vi "Test_LocalQueue Handshake.vi"() -> ()   [LabVIEW 2013]
uses:
  Connection/auth -- cluster.ctl
  <vilib>/LabVIEW Open Source Project/Unicity/RandomStringGenerator/RandomStringGenerator.lvclass
  Connection/Connection.lvclass
panel:
  out "State verfied":bool
  out "Echo":string
  out "Echo verfied":bool
  out "Auth Ack/Nack":string
  out "Challenge verified":bool
  out "error out 2":errorcluster
  out "error out":errorcluster
  out "Client Reader":string
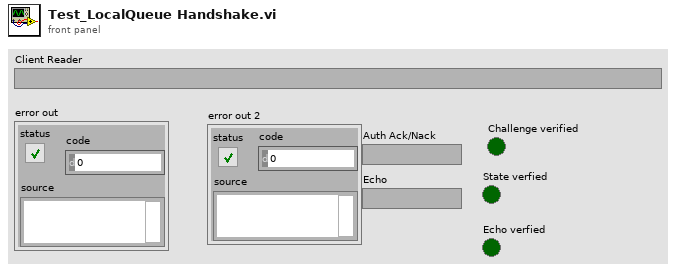
[diagram p1: front panel]
types:
  T1 = typedef "Connection_GOSPL.lvlib/Connection.lvclass/auth -- cluster.ctl" = cluster{"URL":string, "username":string, "state":string}
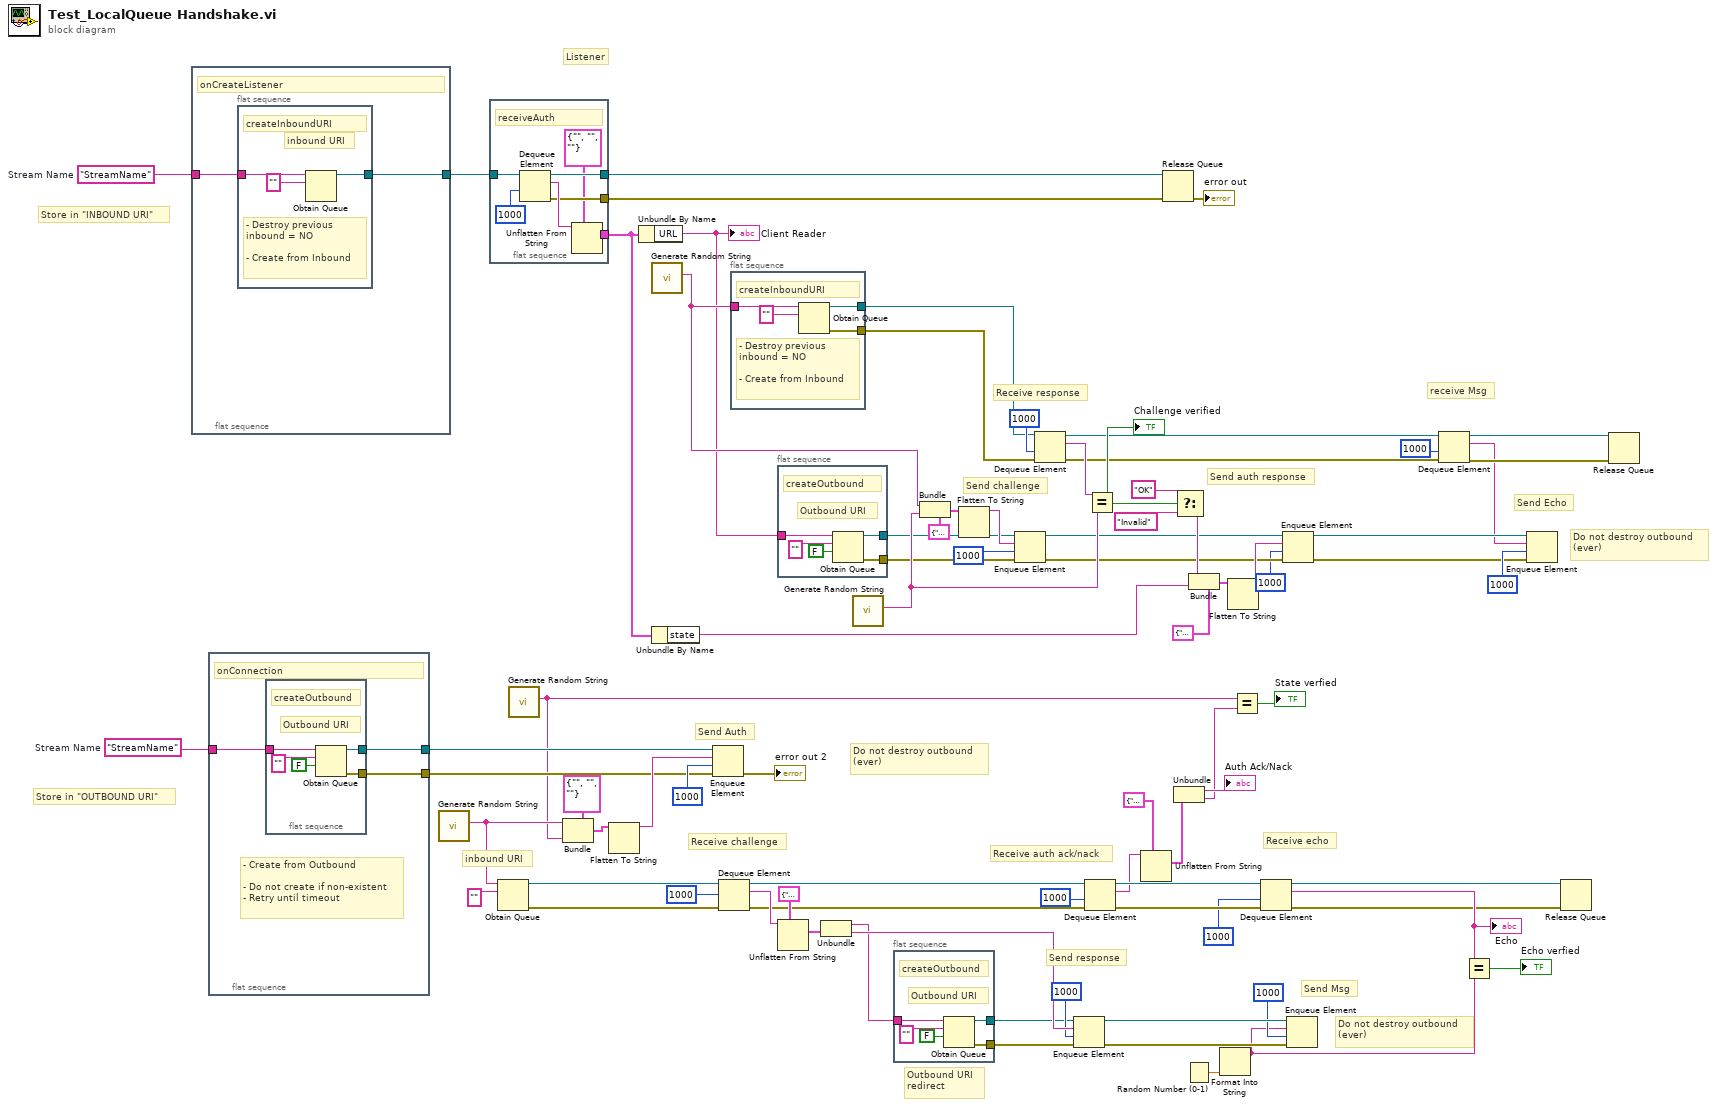
[diagram p0: block diagram]
diagram:
  w59 = "StreamName"  # Stream Name
  w64 = "StreamName"  # Stream Name
  # "Send Msg"
  # "receive Msg"
  # "Store in \"OUTBOUND URI\""
  # "Store in \"INBOUND URI\""
  # "Do not destroy outbound\n(ever)"
  # "Do not destroy outbound\n(ever)"
  # "Do not destroy outbound\n(ever)"
  # "inbound URI"
  # "Listener"
  # "Outbound URI\nredirect"
  # "Send Echo"
  # "Receive echo"
  # "Receive auth ack/nack"
  # "Send auth response"
  # "Receive response"
  # "Send response"
  # "Receive challenge"
  # "Send challenge"
  # "Send Auth"
  n1 = flat-sequence {
    tunnel: w64 -> [w84]
    tunnel: [w83] -> w63
    frame #0 {
      # "onCreateListener"
      n2 = flat-sequence {
        tunnel: w84 -> [w87]
        tunnel: [w85] -> w83
        frame #0 {
          # "- Destroy previous\ninbound = NO\n\n- Create from Inbound"
          # "inbound URI"
          # "createInboundURI"
          n3 = Obtain Queue(name (unnamed)=w87, element data type="") -> (queue out=w85:refnum<queue>)  [unwired: 3 in, 2 out]
        }
      }
    }
  }
  n4 = flat-sequence {
    tunnel: w59 -> [w90]
    tunnel: [w89] -> w56
    tunnel: [w88] -> w53
    frame #0 {
      # "- Create from Outbound\n\n- Do not create if non-existent\n- Retry until timeout"
      # "onConnection"
      n5 = flat-sequence {
        tunnel: w90 -> [w95]
        tunnel: [w93] -> w89
        tunnel: [w92] -> w88
        frame #0 {
          # "Outbound URI"
          # "createOutbound"
          n6 = Obtain Queue(name (unnamed)=w95, element data type="", create if not found? (T)=FALSE) -> (queue out=w93:refnum<queue>, error out=w92:errorcluster)  [unwired: 2 in, 1 out]
        }
      }
    }
  }
  n7 = call <vilib>:"Generate Random String.vi"() -> ("Random String"=w57:string)  [unwired: 11 in]
  n8 = flat-sequence {
    tunnel: [w102] -> w8
    tunnel: w63 -> [w101]
    tunnel: [w98] -> w62
    tunnel: [w97] -> w60
    frame #0 {
      # "receiveAuth"
      n9 = Dequeue Element(queue=w101, timeout in ms (-1)=1000) -> (queue out=w98:refnum<queue>, element=w99:string, error out=w97:errorcluster)  [unwired: 1 in, 1 out]
      n10 = Unflatten From String(type=T1 {"URL"="", "username"="", "state"=""} ("Authorization"), binary string=w99) -> (value=w102:T1)  [unwired: 3 in, 2 out]
    }
  }
  n11 = Obtain Queue(name (unnamed)=w57, element data type="") -> (queue out=w52:refnum<queue>, error out=w50:errorcluster)  [unwired: 3 in, 1 out]
  n12 = call <vilib>:"Generate Random String.vi"() -> ("Random String"=w12:string)  [unwired: 11 in]
  n13 = Bundle(cluster=T1 {"URL"="", "username"="", "state"=""} ("Authorization"), "URL"=w57, "state"=w12) -> (w73:T1)  [unwired: 1 in]
  n14 = Flatten To String(anything=w73) -> (data string=w55:string)  [unwired: 3 in, 2 out]
  n15 = Unbundle By Name(w8) -> ("URL"=w3:string)
  "Client Reader" <- w3
  n16 = call <vilib>:"Generate Random String.vi"() -> ("Random String"=w10:string)  [unwired: 11 in]
  n17 = Unbundle By Name(w8) -> ("state"=w7:string)
  n18 = Enqueue Element(queue=w56, element=w55, timeout in ms (-1)=1000, error in (no error)=w53) -> (error out=→"error out 2":errorcluster)  [unwired: 2 out]
  n19 = Dequeue Element(queue=w52, timeout in ms (-1)=1000, error in (no error)=w50) -> (queue out=w48:refnum<queue>, element=w49:string, error out=w47:errorcluster)  [unwired: 1 out]
  n20 = flat-sequence {
    tunnel: w10 -> [w106]
    tunnel: [w104] -> w11
    tunnel: [w103] -> w9
    frame #0 {
      # "- Destroy previous\ninbound = NO\n\n- Create from Inbound"
      # "createInboundURI"
      n21 = Obtain Queue(name (unnamed)=w106, element data type="") -> (queue out=w104:refnum<queue>, error out=w103:errorcluster)  [unwired: 3 in, 1 out]
    }
  }
  n22 = flat-sequence {
    tunnel: w3 -> [w111]
    tunnel: [w109] -> w2
    tunnel: [w108] -> w1
    frame #0 {
      # "Outbound URI"
      # "createOutbound"
      n23 = Obtain Queue(name (unnamed)=w111, element data type="", create if not found? (T)=FALSE) -> (queue out=w109:refnum<queue>, error out=w108:errorcluster)  [unwired: 2 in, 1 out]
    }
  }
  n24 = Unflatten From String(type=cluster{"redirect":string, "challenge":string} {"redirect"="", "challenge"=""} ("cluster"), binary string=w49) -> (value=w80:cluster{"redirect":string, "challenge":string})  [unwired: 3 in, 2 out]
  n25 = Unbundle(w80) -> ("redirect"=w6:string, "challenge"=w37:string)
  n26 = call <vilib>:"Generate Random String.vi"() -> ("Random String"=w74:string)  [unwired: 11 in]
  n27 = flat-sequence {
    tunnel: w6 -> [w116]
    tunnel: [w114] -> w5
    tunnel: [w113] -> w4
    frame #0 {
      # "Outbound URI"
      # "createOutbound"
      n28 = Obtain Queue(name (unnamed)=w116, element data type="", create if not found? (T)=FALSE) -> (queue out=w114:refnum<queue>, error out=w113:errorcluster)  [unwired: 2 in, 1 out]
    }
  }
  n29 = Bundle(cluster=cluster{"redirect":string, "challenge":string} {"redirect"="", "challenge"=""}, "redirect"=w10, "challenge"=w74) -> (w82:cluster{"redirect":string, "challenge":string})
  n30 = Flatten To String(anything=w82) -> (data string=w23:string)  [unwired: 3 in, 2 out]
  n31 = Enqueue Element(queue=w2, element=w23, timeout in ms (-1)=1000, error in (no error)=w1) -> (queue out=w21:refnum<queue>, error out=w16:errorcluster)  [unwired: 1 out]
  n32 = Dequeue Element(queue=w11, timeout in ms (-1)=1000, error in (no error)=w9) -> (queue out=w28:refnum<queue>, element=w29:string, error out=w24:errorcluster)  [unwired: 1 out]
  n33 = Enqueue Element(queue=w5, element=w37, timeout in ms (-1)=1000, error in (no error)=w4) -> (queue out=w35:refnum<queue>, error out=w32:errorcluster)  [unwired: 1 out]
  n34 = Dequeue Element(queue=w48, timeout in ms (-1)=1000, error in (no error)=w47) -> (queue out=w46:refnum<queue>, element=w41:string, error out=w45:errorcluster)  [unwired: 1 out]
  n35 = Equal?(x=w29, y=w74) -> (x = y?=w79:bool)
  "Challenge verified" <- w79
  n36 = Unflatten From String(type=cluster{"response":string, "header":string} {"response"="", "header"=""} ("cluster"), binary string=w41) -> (value=w68:cluster{"response":string, "header":string})  [unwired: 3 in, 2 out]
  n37 = Release Queue(queue=w62, error in (no error)=w60) -> (error out=→"error out":errorcluster)  [unwired: 1 in, 2 out]
  n38 = Unbundle(w68) -> ("response"=→"Auth Ack/Nack":string, "header"=w66:string)
  n39 = Select(t="OK", s=w79, f="Invalid") -> (s? t:f=w70:string)
  n40 = Random Number (0-1)() -> (number: 0 to 1=w33:dbl)
  n41 = Bundle(cluster=cluster{"response":string, "header":string} {"response"="", "header"=""}, "response"=w70, "header"=w7) -> (w71:cluster{"response":string, "header":string})
  n42 = Format Into String(w33) -> (resulting string=w31:string)  [unwired: 3 in, 1 out]
  n43 = Flatten To String(anything=w71) -> (data string=w17:string)  [unwired: 3 in, 2 out]
  n44 = Equal?(x=w12, y=w66) -> (x = y?=→"State verfied":bool)
  n45 = Dequeue Element(queue=w46, timeout in ms (-1)=1000, error in (no error)=w45) -> (queue out=w40:refnum<queue>, element=w44:string, error out=w39:errorcluster)  [unwired: 1 out]
  "Echo" <- w44
  n46 = Enqueue Element(queue=w21, element=w17, timeout in ms (-1)=1000, error in (no error)=w16) -> (queue out=w19:refnum<queue>, error out=w14:errorcluster)  [unwired: 1 out]
  n47 = Enqueue Element(queue=w35, element=w31, timeout in ms (-1)=1000, error in (no error)=w32) -> ()  [unwired: 3 out]
  n48 = Dequeue Element(queue=w28, timeout in ms (-1)=1000, error in (no error)=w24) -> (queue out=w26:refnum<queue>, element=w18:string, error out=w25:errorcluster)  [unwired: 1 out]
  n49 = Equal?(x=w44, y=w31) -> (x = y?=→"Echo verfied":bool)
  n50 = Enqueue Element(queue=w19, element=w18, timeout in ms (-1)=1000, error in (no error)=w14) -> ()  [unwired: 3 out]
  n51 = Release Queue(queue=w40, error in (no error)=w39) -> ()  [unwired: 1 in, 3 out]
  n52 = Release Queue(queue=w26, error in (no error)=w25) -> ()  [unwired: 1 in, 3 out]
